vi "state_example.vi"(8 "CurrentState":string, 11 "Action":enum16{"Entry", "During", "Exit"}(ring)) -> (0 "NextState":string)   [LabVIEW 2021]
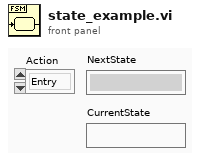
[diagram p1: front panel]
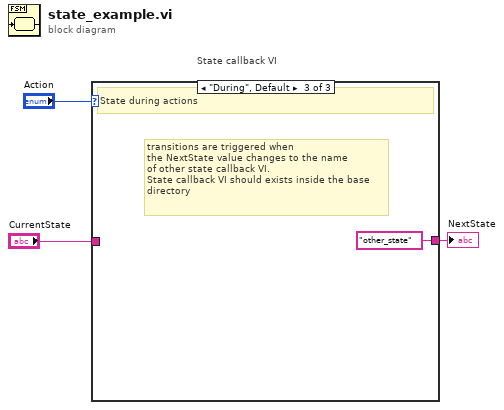
[diagram p0: block diagram]
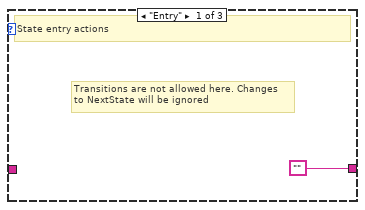
[diagram p2: hidden frame]
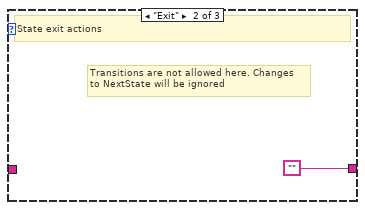
[diagram p3: hidden frame]
diagram:
  # "State callback VI"
  n1 = case shown="\"During\", Default" "Action" {
    tunnel: ["" "" "other_state"] -> w2
    tunnel: "CurrentState" -> [_ _ _]
    frame "Entry" {
      # "Transitions are not allowed here. Changes\nto NextState will be ignored"
      # "State entry actions"
    }
    frame "Exit" {
      # "Transitions are not allowed here. Changes\nto NextState will be ignored"
      # "State exit actions"
    }
    frame "During", Default {
      # "transitions are triggered when\nthe NextState value changes to the name\nof other state callback VI.\nState callback VI should exists inside the base \ndirectory"
      # "State during actions"
    }
  }
  "NextState" <- w2
